vi "Discovery Client FGV.vi"(8 "error in":errorcluster, 11 "action":T2) -> (0 "error out":errorcluster, 3 "grpc client id":T1)   [LabVIEW 2020, in "MeasurementLink Discovery Client Wrapper.lvlib"]
uses:
  MeasurementLink Discovery Client Wrapper.lvlib
  MeasurementLink Measurement Server/MeasurementLink Measurement Server.lvlib
  MeasurementLink Discovery Client/MeasurementLink Discovery Client.lvlib
  <vilib>/gRPC/LabVIEW gRPC Library/Shared/grpcId.ctl
  <vilib>/gRPC/LabVIEW gRPC Library/grpc-lvsupport-release.lvlib
  Action.ctl
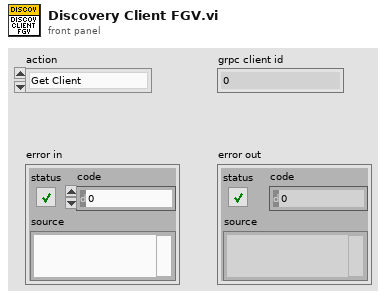
[diagram p1: front panel]
types:
  T1 = typedef "grpc-lvsupport-release.lvlib/grpcId.ctl" = u64
  T2 = typedef "MeasurementLink Discovery Client Wrapper.lvlib/Action.ctl" = enum16{"Get Client", "Destroy Client"}
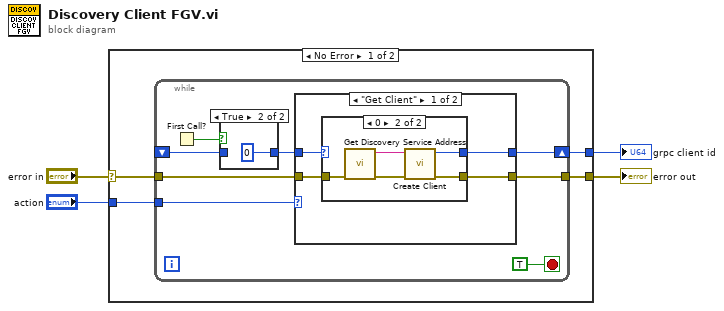
[diagram p0: block diagram]
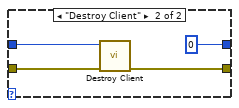
[diagram p4: hidden frame]
diagram:
  n1 = case shown="No Error" "error in" {
    selector: "error in" -> [w7 w34]
    tunnel: [w6 w34] -> w3
    tunnel: "action" -> [w8 _]
    tunnel: [w5 _] -> w1
    frame No Error {
      n2 = while {
        tunnel: w8 -> [w15]
        tunnel: w7 -> [w14]
        shift-right: [w13] -> w5
        shift-left: _ -> [w10]
        tunnel: [w12] -> w6
        stop <- TRUE stop-if-true
        n3 = First Call?() -> (First Call?: T/F=w11:bool)
        n4 = case shown="True" w11 {
          tunnel: w10 -> [w17 _]
          tunnel: [w17 T1 0 ("gRPC ID out")] -> w9
          frame False {
          }
          frame True {
          }
        }
        n5 = case shown="\"Get Client\"" w15 {
          tunnel: w14 -> [w22 w32]
          tunnel: [w20 T1 0 ("gRPC ID out")] -> w13
          tunnel: w9 -> [w21 w33]
          tunnel: [w19 w30] -> w12
          frame "Get Client" {
            n6 = case shown="0" w21 {
              selector: w21 -> [w24 _]
              tunnel: w22 -> [w23 w27]
              tunnel: [w23 w26] -> w19
              tunnel: [w24 w25] -> w20
              frame Default {
              }
              frame 0 {
                n7 = call "Get Discovery Service Address.vi"("error in"=w27) -> ("error out"=w29:errorcluster, "address"=w28:string)  [unwired: 9 in]
                n8 = call "Create Client.vi"("error in"=w29, "address"=w28) -> ("error out"=w26:errorcluster, "gRPC ID Out"=w25:T1)  [unwired: 8 in]
              }
            }
          }
          frame "Destroy Client" {
            n9 = call "Destroy Client.vi"("error in"=w32, "gRPC ID"=w33) -> ("error out"=w30:errorcluster)  [unwired: 9 in]
          }
        }
      }
    }
    frame Error {
    }
  }
  "error out" <- w3
  "grpc client id" <- w1
